vi "Get Unmapped Channels.vi"(8 "error in (no error)":errorcluster, 9 "All Channels":string[](array[string]), 10 "Destinations":string[](array[string]), 11 "Sources":string[](array[string])) -> (0 "error out":errorcluster, 3 "Unmapped Channels":string[](array[string]))   [LabVIEW 2016, in "System Mapping Tool.lvlib"]
uses:
  System Mapping Tool.lvlib
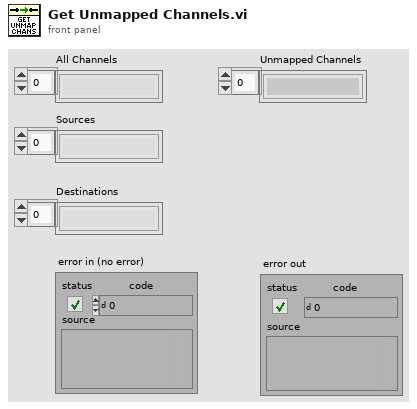
[diagram p1: front panel]
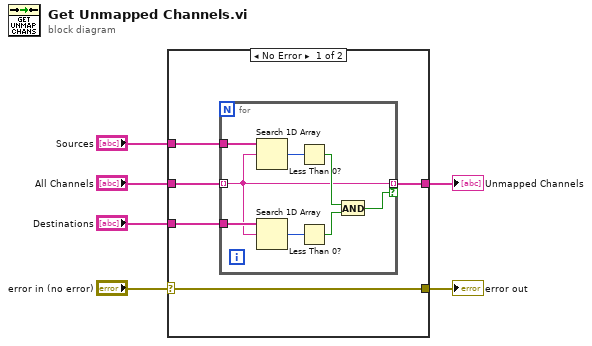
[diagram p0: block diagram]
diagram:
  n1 = case shown="No Error" "error in (no error)" {
    selector: "error in (no error)" -> [w8 w20]
    tunnel: [w8 w20] -> w5
    tunnel: "All Channels" -> [w11 _]
    tunnel: "Sources" -> [w10 _]
    tunnel: "Destinations" -> [w9 _]
    tunnel: [w7 _] -> w1
    frame No Error {
      n2 = for {
        tunnel: w11 -> [w13] mode=indexing
        tunnel: w10 -> [w18]
        tunnel: w9 -> [w19]
        tunnel: [w13] -> w7 mode=indexing if=w12
        n3 = Search 1D Array(1D array=w18, element=w13) -> (index of element=w17:i32)  [unwired: 1 in]
        n4 = Search 1D Array(1D array=w19, element=w13) -> (index of element=w16:i32)  [unwired: 1 in]
        n5 = Less Than 0?(x=w17) -> (x < 0?=w14:bool)
        n6 = Less Than 0?(x=w16) -> (x < 0?=w15:bool)
        n7 = And(x=w14, y=w15) -> (x .and. y?=w12:bool)
      }
    }
    frame Error {
    }
  }
  "error out" <- w5
  "Unmapped Channels" <- w1
